vi "Write SSL Options.vi"(8 "error in (no error)":errorcluster, 10 "Options":T1=50462720 items=["None"=0, "NO_SSLv2|v3|COMPRESSION"=50462720, "SSL_OP_NO_COMPRESSION"=131072, "SSL_OP_NO_SSLv2"=16777216, "SSL_OP_NO_SSLv3"=33554432, "SSL_OP_NO_TLSv1"=67108864, "SSL_OP_NO_TLSv1_2"=134217728, "SSL_OP_NO_TLSv1_1"=268435456], 11 "SSL Client Context in":refnum<class "SSL Client Context.lvclass">) -> (0 "error out":errorcluster, 3 "SSL Client Context out":refnum<class "SSL Client Context.lvclass">)   [LabVIEW 2013, in "OpenSSL Socket.lvlib" / "SSL Client Context.lvclass"]
uses:
  SSL Client Context.lvclass
  SSL_Lib/SSL-Context/SSL Options.ctl
  SSL Client Context.lvclass/SSL Client Context.ctl
  SSL_Lib/SSL-Context/SSL-Context.lvclass
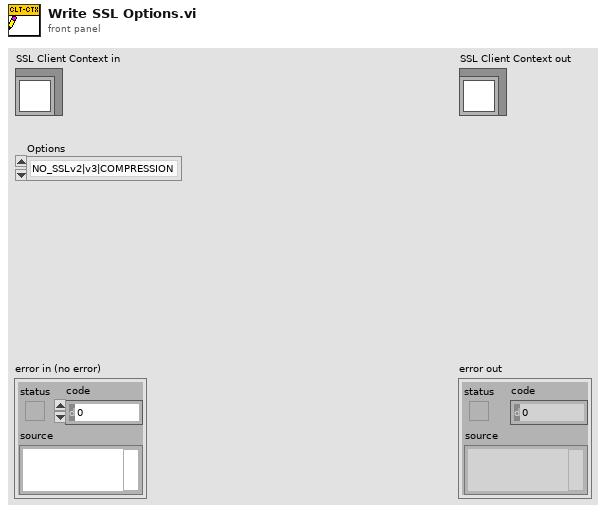
[diagram p1: front panel]
types:
  T1 = typedef "SSL_Lib.lvlib/SSL-Context.lvclass/SSL Options.ctl" = i32
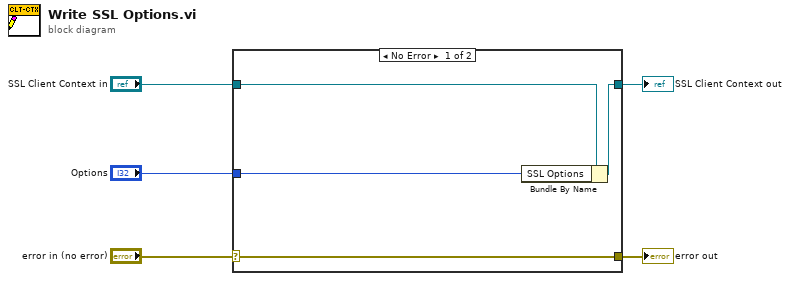
[diagram p0: block diagram]
diagram:
  n1 = case shown="No Error" "error in (no error)" {
    selector: "error in (no error)" -> [w9 w10]
    tunnel: [w9 w10] -> w4
    tunnel: [w7 w11] -> w2
    tunnel: "SSL Client Context in" -> [w8 w11]
    tunnel: "Options" -> [w6 _]
    frame No Error {
      n2 = Bundle By Name(cluster=w8, "SSL Options"=w6) -> (w7:refnum<class "SSL Client Context.lvclass">)
    }
    frame Error {
    }
  }
  "error out" <- w4
  "SSL Client Context out" <- w2
